vi "stop_all_axes.vi"(11 "VISA Refnum in":refnum<visa-resource-name>) -> ()   [LabVIEW 2025]
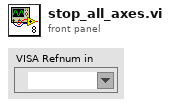
[diagram p1: front panel]
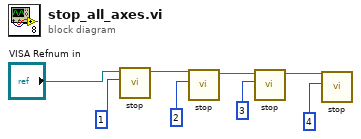
[diagram p0: block diagram]
diagram:
  n1 = call "stop.vi"("Axis in"=1, "VISA Handle in"="VISA Refnum in") -> ("VISA Handle out"=w6:refnum<visa-resource-name>)  [unwired: 4 in, 3 out]
  n2 = call "stop.vi"("Axis in"=2, "VISA Handle in"=w6) -> ("VISA Handle out"=w5:refnum<visa-resource-name>)  [unwired: 4 in, 3 out]
  n3 = call "stop.vi"("Axis in"=3, "VISA Handle in"=w5) -> ("VISA Handle out"=w4:refnum<visa-resource-name>)  [unwired: 4 in, 3 out]
  n4 = call "stop.vi"("Axis in"=4, "VISA Handle in"=w4) -> ()  [unwired: 4 in, 4 out]
